vi "SimpleEvents.vi"() -> ()   [LabVIEW 2011]
uses:
  <vilib>/Platform/TimedLoop/XDataNode/timing_clust.ctl
  <vilib>/Platform/TimedLoop/XDataNode/nitl_modes.ctl
  <vilib>/Platform/TimedLoop/XDataNode/wakeup.ctl
  <vilib>/Platform/TimedLoop/XDataNode/XDataNode.xnode
  <vilib>/Platform/TimedLoop/XDataNode/XDNodeRunTimeDep.lvlib
panel:
  out "Time Stamp":timestamp
  out "Waveform Chart":dbl(graph)
  in  "stop":bool
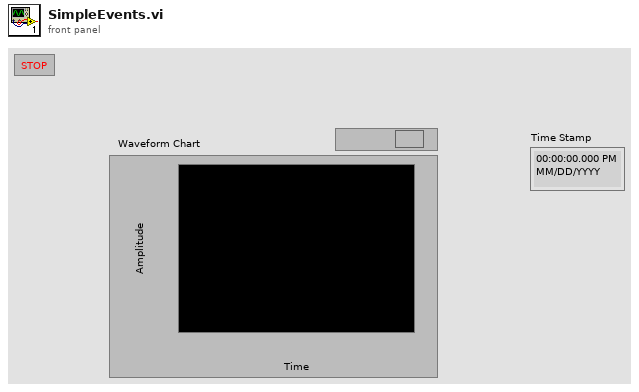
[diagram p1: front panel]
types:
  T1 = typedef "XDNodeRunTimeDep.lvlib/timing_clust.ctl" = cluster{"Expected End [f-1]":u64, "Actual End [f-1]":u64, "Finished Late? [f-1]":bool, "Expected End [i-1]":u64, "Actual End [i-1]":u64, "Finished Late? [i-1]":bool, "Expected Start [i]":u64, "Actual Start [i]":u64, "Expected Start [f]":u64, "Actual Start [f]":u64, "Source Name":string, "Structure Name":string, "Period":i64, "Deadline":i64, "Offset":i64, "Start":i64, "Priority":i32, "Timeout":i32, "Mode":T2, "Wakeup Reason":T3, "Error":errorcluster, "Source Type":string, "Secondary Source Type":string, "Global End Time":u64, "Global Start Time":u64, "Frame Duration":u64, "Iteration Duration":u64, "Assigned CPU":i32, "I/O Scan Engine Mode":u32}
  T2 = typedef "XDNodeRunTimeDep.lvlib/nitl_modes.ctl" = enum32{"No Change", "Process missed periods, maintain original phase", "Discard missed periods, maintain original phase", "Process missed periods, ignore original phase", "Discard missed periods, ignore original phase"}
  T3 = typedef "XDNodeRunTimeDep.lvlib/wakeup.ctl" = enum32{"Normal", "Aborted", "Asynchronous wakeup", "Timing source error", "Timed loop error", "Timeout"}
  T4 = cluster{"seconds since 1Jan1904":timestamp, "number: 0 to 1":dbl}
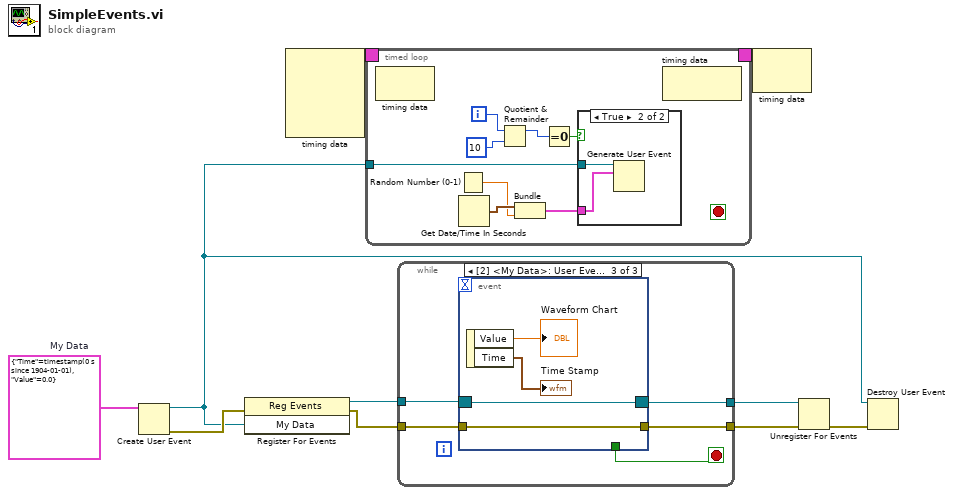
[diagram p0: block diagram]
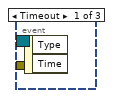
[diagram p3: hidden frame]
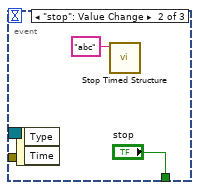
[diagram p4: hidden frame]
diagram:
  w9 = cluster{"Time":timestamp, "Value":dbl} {"Time"=timestamp(0 s since 1904-01-01), "Value"=0.0}  # My Data
  n1 = Create User Event(user event datatype=w9) -> (user event=w1:refnum<user-event>, error out=w10:errorcluster)  [unwired: 1 in]
  n2 = register-events(error in=w10, w1) -> (reference out=w8:refnum<event-registration>, error out=w5:errorcluster)  [unwired: 1 in]
  n3 = node-c288() -> (w7:T1)  [unwired: 4 in]
  n4 = timed-loop {
    timing: w7 -> [_]
    timing-out: [_] -> w6
    tunnel: w1 -> [w18]
    i -> [w17]
    stop <- _ stop-if-true
    n5 = node-c288() -> ()  [unwired: 1 in, 1 out]
    n6 = Random Number (0-1)() -> (number: 0 to 1=w11:dbl)
    n7 = Get Date/Time In Seconds() -> (seconds since 1Jan1904=w12:timestamp)
    n8 = Quotient & Remainder(x=w17, y=10 ("x")) -> (x-y*floor(x/y)=w14:i32)  [unwired: 1 out]
    n9 = Bundle("seconds since 1Jan1904"=w12, "number: 0 to 1"=w11) -> (w13:T4)  [unwired: 1 in]
    n10 = Equal To 0?(x=w14) -> (x = 0?=w15:bool)
    n11 = case shown="True" w15 {
      tunnel: w18 -> [_ w20]
      tunnel: w13 -> [_ w19]
      frame False {
      }
      frame True {
        n12 = Generate User Event(user event=w20, event data cluster=w19) -> ()  [unwired: 1 in, 2 out]
      }
    }
    n13 = node-c288() -> ()  [unwired: 1 in, 1 out]
  }
  n14 = while {
    tunnel: w8 -> [w27]
    tunnel: [w26] -> w3
    tunnel: w5 -> [w25]
    tunnel: [w24] -> w4
    stop <- w23 stop-if-true
    n15 = event shown="[2] <My Data>: User Event" {
      selector: w27 -> [_ _ w31]
      dyn-events: [_ _ w31] -> w26
      timeout: _ -> [_ _ _]
      tunnel: w25 -> [_ _ w30]
      tunnel: [_ _ w30] -> w24
      tunnel: [_ "stop" _] -> w23
      event Timeout {
        n16 = event-data() -> ()  [unwired: 1 in, 2 out]
      }
      event "stop": Value Change {
        n17 = event-data() -> ()  [unwired: 1 in, 2 out]
        n18 = call <vilib>:"Stop Timed Structure.vi"("name"="abc") -> ()  [unwired: 10 in, 1 out]
      }
      event User Event {
        n19 = event-data() -> ("Value"=→"Waveform Chart":dbl, "Time"=→"Time Stamp":timestamp)  [unwired: 1 in]
      }
    }
  }
  n20 = node-c288(w6) -> ()  [unwired: 1 out]
  n21 = Unregister For Events(event registration refnum=w3, error in=w4) -> (error out=w2:errorcluster)
  n22 = Destroy User Event(user event=w1, error in=w2) -> ()  [unwired: 1 out]
